vi "CW Steps Selected.vi"(8 "error in":errorcluster, 11 "Wash Options":T1) -> (0 "error out":errorcluster, 3 "Car Wash Steps":string[][](array[string]))   [LabVIEW 2020]
uses:
  Controls/Wash Options.ctl
  <vilib>/Utility/file.llb/Read Delimited Spreadsheet (string).vi
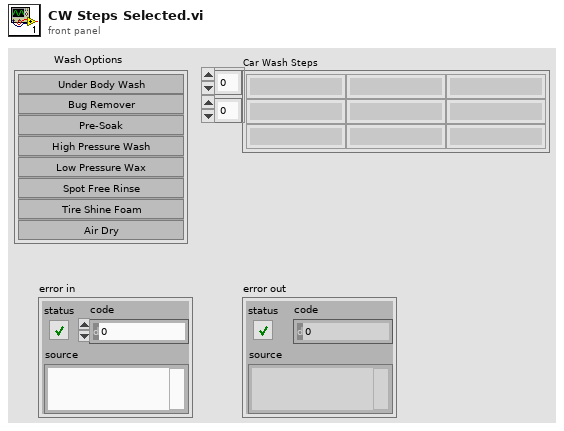
[diagram p1: front panel]
types:
  T1 = typedef "Wash Options.ctl" = cluster{"Underbody Wash":bool, "Bug Remover":bool, "Pre-Soak":bool, "High Pressure Wash":bool, "Low Pressure Wax":bool, "Spot Free Rinse":bool, "Tire Shine Foam":bool, "Air Dry":bool}
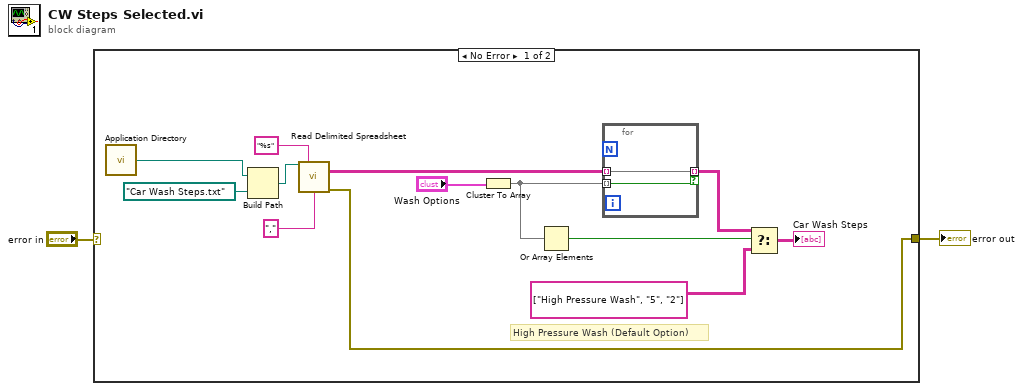
[diagram p0: block diagram]
diagram:
  n1 = case shown="No Error" "error in" {
    selector: "error in" -> [_ w18]
    tunnel: [w9 w18] -> w2
    frame No Error {
      # "High Pressure Wash (Default Option)"
      n2 = call <vilib>:"Application Directory.vi"() -> ("Application Directory"=w13:path)
      n3 = Build Path(base path=w13, name or relative path=path "Car Wash Steps.txt" ("file path (dialog if empty)")) -> (appended path=w14:path)
      n4 = call-poly <vilib>:"Read Delimited Spreadsheet.vi"("file path (dialog if empty)"=w14, "format (%s)"="%s" ("format (%.3f)"), "delimiter (\\t)"="," ("delimiter (\\t)")) -> ("all rows"=w4:string[][], "error out"=w9:errorcluster)  [unwired: 7 in, 4 out]
      n5 = Cluster To Array(cluster="Wash Options") -> (array=w8:bool[])
      n6 = Or Array Elements(Boolean array=w8) -> (logical OR=w7:bool)
      n7 = for {
        tunnel: w4 -> [w17] mode=indexing
        tunnel: [w17] -> w6 mode=indexing if=w16
        tunnel: w8 -> [w16] mode=indexing
      }
      n8 = Select(t=w6, s=w7, f=string[][] [["High Pressure Wash", "5", "2"]] ("all rows")) -> (s? t:f=→"Car Wash Steps":string[][])
    }
    frame Error {
    }
  }
  "error out" <- w2
